vi "construct_sensitivity_tf_cd.vi"(5 "ki":dbl, 6 "K":dbl, 7 "kp":dbl, 8 "wf":dbl, 9 "h":dbl, 10 "tau":dbl) -> (0 "error out":errorcluster, 1 "C(s)":T1 {"transfer function(s)"."delay" format="%.4f"; "transfer function(s)"."Denominator" format="%#_3g"; "transfer function(s)"."Numerator" format="%#_3g"; "properties"."Sampling Time" format="%#.6p"; "properties"."Output Delays" format="%.4f"; "properties"."Input Delays" format="%.4f"}, 2 "L(s)":T1 {"transfer function(s)"."delay" format="%.4f"; "transfer function(s)"."Denominator" format="%#_3g"; "transfer function(s)"."Numerator" format="%#_3g"; "properties"."Sampling Time" format="%#.6p"; "properties"."Output Delays" format="%.4f"; "properties"."Input Delays" format="%.4f"}, 3 "P(s)":T1 {"transfer function(s)"."delay" format="%.4f"; "transfer function(s)"."Denominator" format="%#_3g"; "transfer function(s)"."Numerator" format="%#_3g"; "properties"."Sampling Time" format="%#.6p"; "properties"."Output Delays" format="%.4f"; "properties"."Input Delays" format="%.4f"}, 4 "S(s)":T1 {"transfer function(s)"."delay" format="%.4f"; "transfer function(s)"."Denominator" format="%#_3g"; "transfer function(s)"."Numerator" format="%#_3g"; "properties"."Sampling Time" format="%#.6p"; "properties"."Output Delays" format="%.4f"; "properties"."Input Delays" format="%.4f"})   [LabVIEW 2021]
doc: "Consturct the sensitivity transfer function of a first-order plant with filtering and sampling delay."
uses:
  <vilib>/addons/Control Design/_Model Construction/Model Typedefs.llb/CD Transfer Function Model (MIMO).ctl
  <vilib>/addons/Control Design/_Model Construction/Model Typedefs.llb/CD General Elements.ctl
  <vilib>/addons/Control Design/_Model Construction/Model Typedefs.llb/CD Transfer Function Model (SISO).ctl
  <vilib>/addons/Control Design/_Model Construction/Special Model Creation.llb/Special Model Creation SubVI/CD Create 1st Order Model.vi
  <vilib>/addons/Control Design/_Model Interconnection/Model Interconnection.llb/Model Interconnection SubVI/cd_Series (TF and TF).vi
  <vilib>/addons/Control Design/_Model Construction/Special Model Creation.llb/Special Model Creation SubVI/CD Create PID Parallel Model.vi
  <vilib>/addons/Control Design/_Model Delay/Model Delay.llb/Model Delay subVIs/cd_Convert Delay with Pade Approx (TF).vi
  <vilib>/addons/Control Design/_Model Interconnection/Model Interconnection.llb/Model Interconnection SubVI/cd_Feedback (TF and TF).vi
  <vilib>/addons/Control Design/_Model Construction/NI_CD_Special Model Creation.lvlib
  <vilib>/addons/Control Design/_Model Interconnection/NI_CD_Model Interconnection.lvlib
  <vilib>/addons/Control Design/_Model Delay/NI_CD_Model Delay.lvlib
  <vilib>/addons/Control Design/_Model Construction/NI_LinSys_Model Typedefs.lvlib
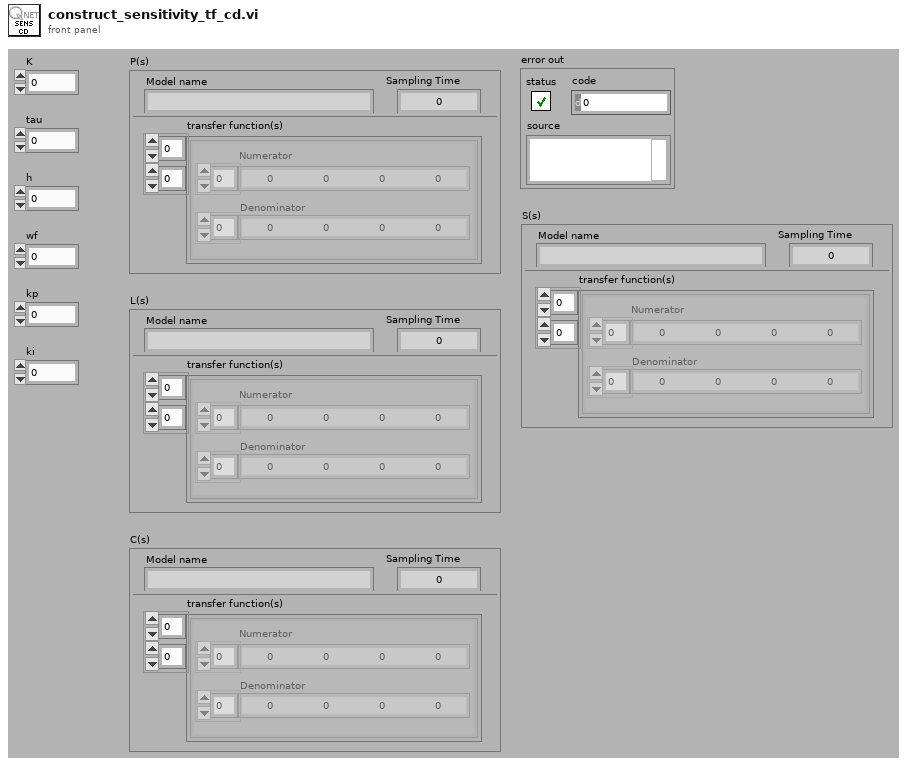
[diagram p1: front panel]
types:
  T1 = typedef "NI_LinSys_Model Typedefs.lvlib/CD Transfer Function Model (MIMO).ctl" = cluster{"properties":T2, "transfer function(s)":T3[][]}
  T2 = typedef "NI_LinSys_Model Typedefs.lvlib/CD General Elements.ctl" = cluster{"Model name":string, "Input names":string[], "Output names":string[], "Input Delays":dbl[], "Output Delays":dbl[], "Sampling Time":dbl, "Notes":string}
  T3 = typedef "NI_LinSys_Model Typedefs.lvlib/CD Transfer Function Model (SISO).ctl" = cluster{"Numerator":dbl[], "Denominator":dbl[], "delay":dbl}
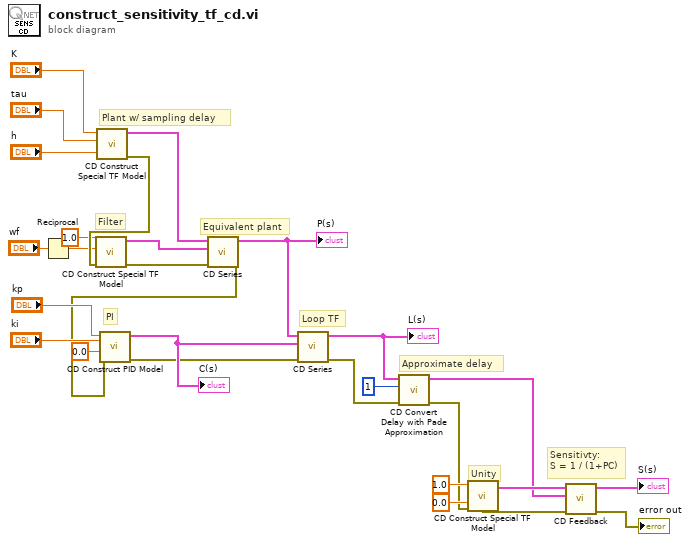
[diagram p0: block diagram]
diagram:
  # "Equivalent plant"
  # "Sensitivty:\nS = 1 / (1+PC)"
  # "Loop TF"
  # "Approximate delay"
  # "Unity"
  # "PI"
  # "Filter"
  # "Plant w/ sampling delay"
  n1 = Reciprocal(x="wf") -> (1/x=w3:dbl)
  n2 = call-poly <vilib>:"CD Construct Special TF Model.vi"("Delay"="h", "Time Constant (s)"="tau", "Static Gain"="K") -> ("error out"=w14:errorcluster, "Transfer Function Model"=w12:T1)  [unwired: 1 in, 6 out]
  n3 = call-poly <vilib>:"CD Construct Special TF Model.vi"("error in (no error)"=w14, "Time Constant (s)"=w3, "Static Gain"=1.0) -> ("error out"=w15:errorcluster, "Transfer Function Model"=w13:T1)  [unwired: 1 in, 6 out]
  n4 = call-poly <vilib>:"CD Series.vi"("error in (no error)"=w15, "Model 2"=w13, "Model 1"=w12) -> ("error out"=w2:errorcluster, "Series Model"=w26:T1)  [unwired: 7 out]
  "P(s)" <- w26
  n5 = call-poly <vilib>:"CD Construct PID Model.vi"("error in (no error)"=w2, "Derivative Gain (Kd)"=0.0, "Integral Gain (Ki)"="ki", "Proportional Gain (Kp)"="kp") -> ("error out"=w1:errorcluster, "Transfer Function Model"=w28:T1)  [unwired: 1 in, 5 out]
  "C(s)" <- w28
  n6 = call-poly <vilib>:"CD Series.vi"("error in (no error)"=w1, "Model 2"=w28, "Model 1"=w26) -> ("error out"=w6:errorcluster, "Series Model"=w27:T1)  [unwired: 7 out]
  "L(s)" <- w27
  n7 = call-poly <vilib>:"CD Convert Delay with Pade Approximation.vi"("error in (no error)"=w6, "Polynomial Order"=1, "Transfer Function Model"=w27) -> ("error out"=w5:errorcluster, "Transfer Function Converted Model"=w22:T1)  [unwired: 7 out]
  n8 = call-poly <vilib>:"CD Construct Special TF Model.vi"("error in (no error)"=w5, "Time Constant (s)"=0.0, "Static Gain"=1.0) -> ("error out"=w4:errorcluster, "Transfer Function Model"=w23:T1)  [unwired: 1 in, 6 out]
  n9 = call-poly <vilib>:"CD Feedback.vi"("error in (no error)"=w4, "Model 2"=w22, "Model 1"=w23) -> ("error out"=→"error out":errorcluster, "Closed-Loop Model"=→"S(s)":T1)  [unwired: 1 in, 6 out]
